vi "Configure Trigger (Edge).vi"(0 "VISA resource name":refnum<visa-resource-name>, 5 "Trigger Source (0: Channel 1)":i32(ring) items=["Channel 1", "Channel 2", "Channel 3", "Channel 4", "External Input", "Attenuated External Input"], 7 "Trigger Level (0.0 V)":dbl, 9 "Trigger Mode (0: Auto)":i32(ring) items=["Auto", "Normal"], 11 "error in (no error)":errorcluster, 12 "Holdoff (0.00)":dbl format="%_3g", 13 "Trigger Slope (0: Rising)":i32(ring) items=["Rising", "Falling"], 14 "Trigger Coupling (0: AC)":i32(ring) items=["AC", "DC", "HF Reject", "LF Reject", "Noise Reject"]) -> (4 "VISA resource name out":refnum<visa-resource-name>, 15 "error out":errorcluster)   [LabVIEW 2017, in "Tektronix TDS 200 1000 2000 Series.lvlib"]
doc: "Configures edge trigger settings. An edge trigger occurs when the trigger signal passes through the voltage threshold that you specify with the <B>Trigger Level</B> control and has the slope that you specify with the <B>Trigger Slope</B> control. \n\n<b>Note(s):</b>\nUse Wait for Triggered Acquisition.vi before Read Waveform to wait for trigger to happen before acquiring any waveform."
uses:
  Tektronix TDS 200 1000 2000 Series.lvlib
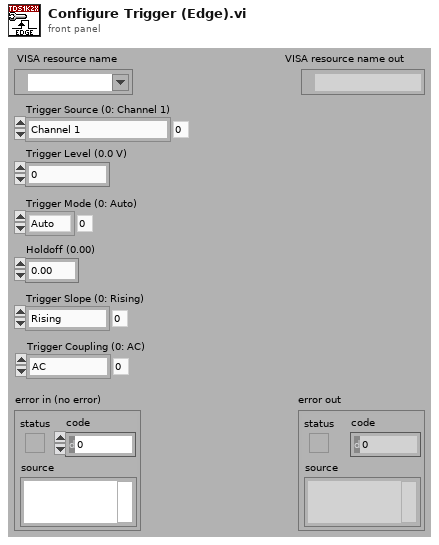
[diagram p1: front panel]
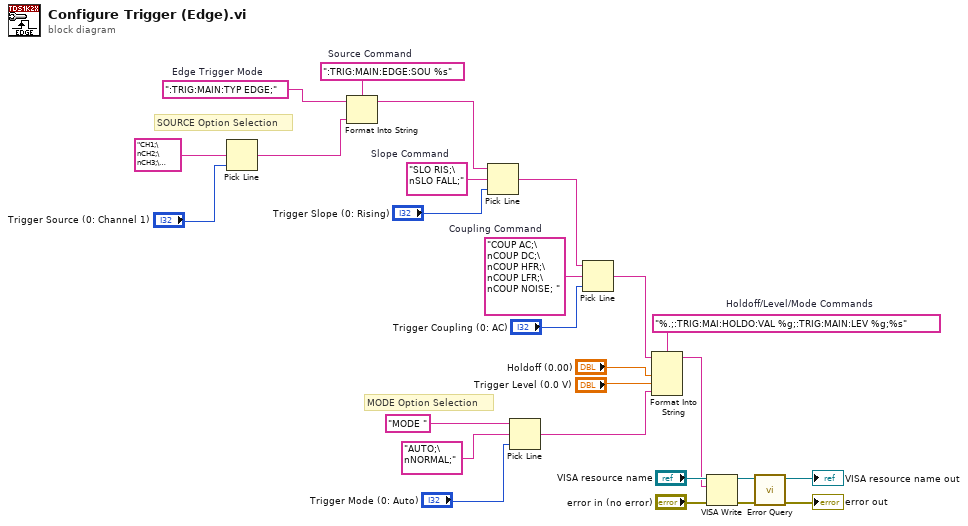
[diagram p0: block diagram]
diagram:
  w4 = "COUP AC;\nCOUP DC;\nCOUP HFR;\nCOUP LFR;\nCOUP NOISE; "  # Coupling Command
  w17 = "SLO RIS;\nSLO FALL;"  # Slope Command
  w18 = "%.;:TRIG:MAI:HOLDO:VAL %g;:TRIG:MAIN:LEV %g;%s"  # Holdoff/Level/Mode Commands
  w19 = ":TRIG:MAIN:TYP EDGE;"  # Edge Trigger Mode
  w20 = ":TRIG:MAIN:EDGE:SOU %s"  # Source Command
  # "MODE Option Selection"
  # "SOURCE Option Selection"
  n1 = Pick Line(multi-line string="CH1;\nCH2;\nCH3;\nCH4;\nEXT;\nEXT5;", line index="Trigger Source (0: Channel 1)") -> (output string=w11:string)  [unwired: 1 out]
  n2 = Format Into String(format string=w20, initial string=w19, w11) -> (resulting string=w14:string)  [unwired: 1 in, 1 out]
  n3 = Pick Line(string ("")=w14, multi-line string=w17, line index="Trigger Slope (0: Rising)") -> (output string=w2:string)
  n4 = Pick Line(string ("")="MODE ", multi-line string="AUTO;\nNORMAL;", line index="Trigger Mode (0: Auto)") -> (output string=w7:string)
  n5 = Pick Line(string ("")=w2, multi-line string=w4, line index="Trigger Coupling (0: AC)") -> (output string=w1:string)
  n6 = Format Into String(format string=w18, initial string=w1, "Holdoff (0.00)", "Trigger Level (0.0 V)", w7) -> (resulting string=w15:string)  [unwired: 1 in, 1 out]
  n7 = VISA Write(VISA resource name="VISA resource name", write buffer=w15, error in (no error)="error in (no error)") -> (VISA resource name out=w22:refnum<visa-resource-name>, error out=w21:errorcluster)  [unwired: 1 out]
  n8 = call "Error Query.vi"("error in (no error)"=w21, "VISA resource name"=w22) -> ("error out"=→"error out":errorcluster, "VISA resource name out"=→"VISA resource name out":refnum<visa-resource-name>)  [unwired: 8 out]
